vi "Read pOriginY.vi"(8 "error in (no error)":errorcluster, 11 "POrigin in":refnum<class "POrigin.lvclass">) -> (0 "error out":errorcluster, 2 "pOriginY":dbl[unit] min=-0.1 max=0.1, 3 "POrigin out":refnum<class "POrigin.lvclass">)   [LabVIEW 2022 SP3, in "TCSDataDefinitions.lvlib" / "TCSCommand.lvlib" / "POriginCommands.lvlib" / "POrigin.lvclass"]
uses:
  POrigin.lvclass
  POrigin.lvclass/POrigin.ctl
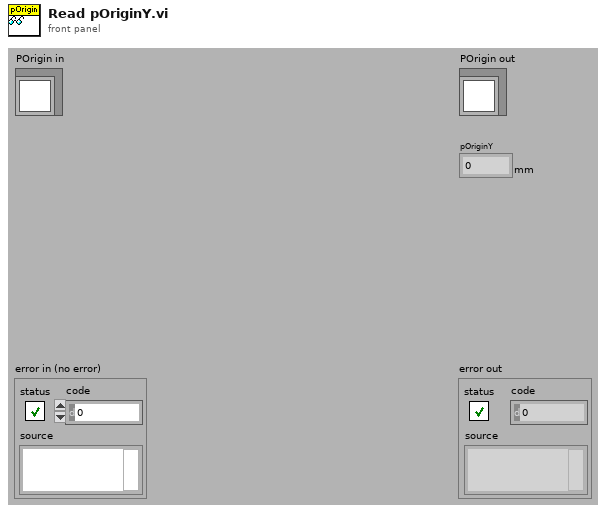
[diagram p1: front panel]
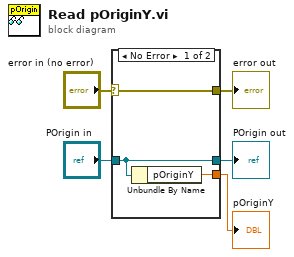
[diagram p0: block diagram]
diagram:
  n1 = case shown="No Error" "error in (no error)" {
    selector: "error in (no error)" -> [w8 w9]
    tunnel: [w8 w9] -> w4
    tunnel: [w7 w10] -> w2
    tunnel: "POrigin in" -> [w7 w10]
    tunnel: [w6 _] -> w1
    frame No Error {
      n2 = Unbundle By Name(w7) -> ("pOriginY"=w6:dbl[unit])
    }
    frame Error {
    }
  }
  "error out" <- w4
  "POrigin out" <- w2
  "pOriginY" <- w1
